vi "Write Name.vi"(10 "Name":string, 11 "Game Board Component in":refnum<class "Game Board Component.lvclass">) -> (3 "Game Board Component out":refnum<class "Game Board Component.lvclass">)   [LabVIEW 2024, in "Game Board Component.lvclass"]
doc: "MIT Licence\nCopyright (c) 2024 David Grollier"
uses:
  Game Board Component.lvclass
  Game Board Component.lvclass/Game Board Component.ctl
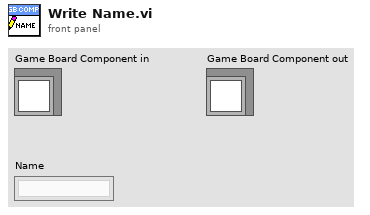
[diagram p1: front panel]
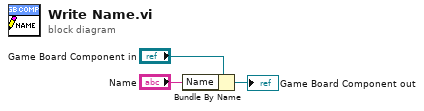
[diagram p0: block diagram]
diagram:
  n1 = Bundle By Name(cluster="Game Board Component in", "Name"="Name") -> (→"Game Board Component out":refnum<class "Game Board Component.lvclass">)
